vi "sanitize tag.vi"(11 "tag descriptor":refnum<class "tag descriptor.lvclass">) -> (3 "clean tag":refnum<class "tag descriptor.lvclass">)   [LabVIEW 2013, in "engine configuration.lvclass"]
uses:
  engine configuration.lvclass
  <vilib>/NI/Tag Bus/tag/tag descriptor.lvclass
  <vilib>/NI/Tag Bus/tag/tag descriptor.lvclass/tag descriptor.ctl
  <vilib>/NI/Tag Bus/tag/read metadata.vi
  <vilib>/NI/Tag Bus/tag/read tag name.vi
  <vilib>/NI/Tag Bus/tag/read data type.vi
  <vilib>/NI/Tag Bus/tag/read raw default value.vi
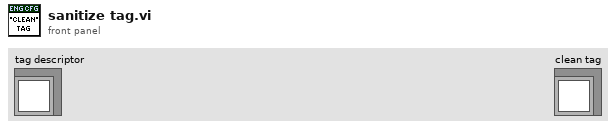
[diagram p1: front panel]
types:
  T1 = typedef "tag bus.lvlib/tag descriptor.lvclass/Data Type.ctl" = enum16{"Double", "Single", "I64", "I32", "I16", "I8", "U64", "U32", "U16", "U8", "Boolean", "String", "Array of Double", "Array of Single", "Array of I64", "Array of I32", "Array of I16", "Array of I8", "Array of U64", "Array of U32", "Array of U16", "Array of U8", "Array of Boolean", "Array of String"}
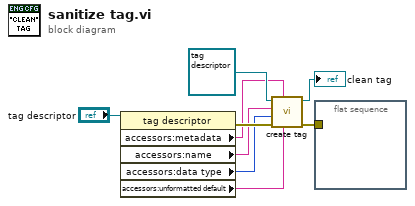
[diagram p0: block diagram]
diagram:
  n1 = property class="tag descriptor"(reference="tag descriptor") -> (error out=w5:errorcluster, "accessors:metadata"=w4:string, "accessors:name"=w1:string, "accessors:data type"=w2:T1, "accessors:unformatted default"=w3:string)  [unwired: 1 in, 1 out]
  n2 = call-dynamic "create tag.vi"("raw default"=w3, "metadata"=w4, "error in"=w5, "data type"=w2, "name"=w1, "tag descriptor in"=refnum<class "tag descriptor.lvclass"> refnum ("tag descriptor")) -> ("error out"=w7:errorcluster, "tag descriptor out"=→"clean tag":refnum<class "tag descriptor.lvclass">)  [unwired: 4 in]
  n3 = flat-sequence {
    tunnel: w7 -> [_]
    frame #0 {
    }
  }
